vi "Abort Acquisition.vi"(8 "error in (no error)":errorcluster, 11 "CCDCamera in":refnum<class "Sim_CCD.lvclass">) -> (0 "error out":errorcluster, 3 "CCDCamera out":refnum<class "Sim_CCD.lvclass">)   [LabVIEW 2018, in "Sim_CCD.lvclass"]
doc: "Abort current acquisition"
uses:
  Sim_CCD.lvclass
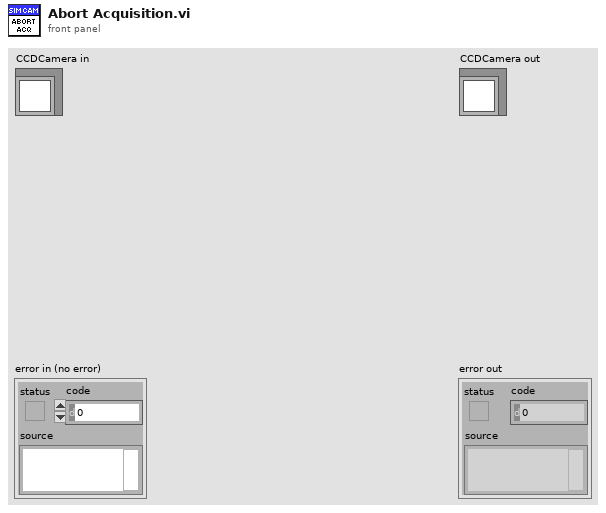
[diagram p1: front panel]
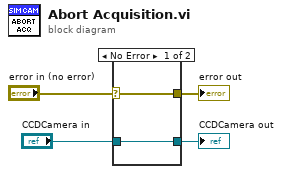
[diagram p0: block diagram]
diagram:
  n1 = case shown="No Error" "error in (no error)" {
    selector: "error in (no error)" -> [w5 w7]
    tunnel: [w5 w7] -> w3
    tunnel: "CCDCamera in" -> [w6 w8]
    tunnel: [w6 w8] -> w2
    frame No Error {
    }
    frame Error {
    }
  }
  "error out" <- w3
  "CCDCamera out" <- w2
